vi "MFC W R.vi"() -> ()   [LabVIEW 2011]
uses:
  <vilib>/rvi/eio/common/nirviEmuTemplateMethod_errors.vi
  <vilib>/eio/EIOMethodNode/EIOMethodNode.xnode
panel:
  out "Array":u32[](array[numeric])
  out "Total time":u32
  in  "Array 1 MFC 2":i16[](array[numeric])=[0, 0]
  out "Array Out":u8[](array[numeric])
  in  "Array 1 MFC":i16[](array[numeric])=[0, 0, 0, 0, 0, 0, 0]
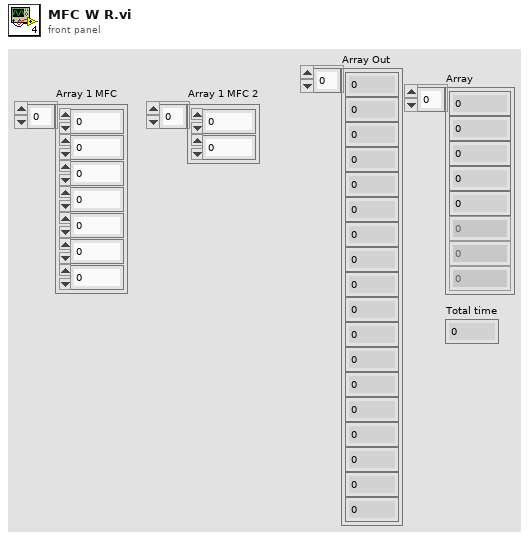
[diagram p1: front panel]
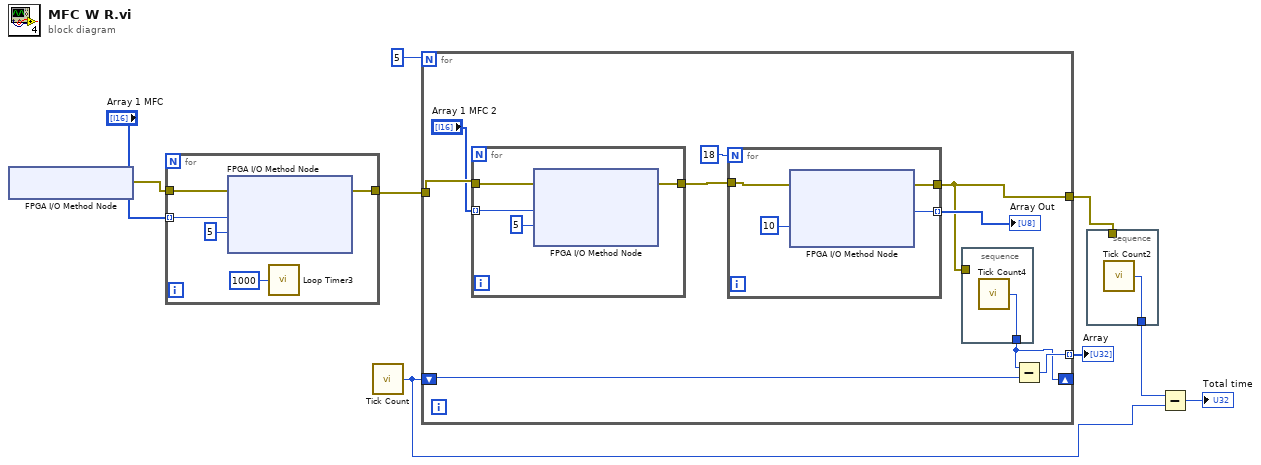
[diagram p0: block diagram]
diagram:
  n1 = xnode "FPGA I/O Method Node"() -> ("error out"=w9:errorcluster)  [unwired: 2 in, 1 out]
  n2 = for {
    tunnel: "Array 1 MFC" -> [w13] mode=indexing
    tunnel: [w11] -> w8
    tunnel: w9 -> [w10]
    n3 = xnode "FPGA I/O Method Node"("error in"=w10, "Data"=w13, "Timeout (ms)"=5) -> ("error out"=w11:errorcluster)  [unwired: 1 in, 2 out]
    n4 = call "Loop Timer3"("Count(uSec)"=u32 1000) -> ()  [unwired: 1 out]
  }
  n5 = call "Tick Count"() -> ("Tick Count(uSec)"=w5:u32)
  n6 = for {
    N: i16 5 -> [_]
    tunnel: w8 -> [w20]
    tunnel: [w18] -> w2
    shift-right: [w15] -> _
    shift-left: w5 -> [w17]
    tunnel: [w16] -> w1 mode=indexing
    n7 = for {
      tunnel: "Array 1 MFC 2" -> [w31] mode=indexing
      tunnel: [w30] -> w22
      tunnel: w20 -> [w29]
      n8 = xnode "FPGA I/O Method Node"("error in"=w29, "Data"=w31, "Timeout (ms)"=5) -> ("error out"=w30:errorcluster)  [unwired: 1 in, 2 out]
    }
    n9 = for {
      N: 18 -> [_]
      tunnel: w22 -> [w27]
      tunnel: [w26] -> w23 mode=indexing
      tunnel: [w25] -> w18
      n10 = xnode "FPGA I/O Method Node"("error in"=w27, "Timeout (ms)"=10) -> ("error out"=w25:errorcluster, "Data"=w26:u8)  [unwired: 1 in, 2 out]
    }
    "Array Out" <- w23
    n11 = stacked-sequence {
      tunnel: [w24] -> w15
      tunnel: w18 -> [_]
      frame #0 {
        n12 = call "Tick Count4"() -> ("Tick Count(uSec)"=w24:u32)
      }
    }
    n13 = Subtract(x=w15, y=w17) -> (x-y=w16:u32)
  }
  "Array" <- w1
  n14 = stacked-sequence {
    tunnel: [w33] -> w3
    tunnel: w2 -> [_]
    frame #0 {
      n15 = call "Tick Count2"() -> ("Tick Count(uSec)"=w33:u32)
    }
  }
  n16 = Subtract(x=w3, y=w5) -> (x-y=→"Total time":u32)
